vi "UI Error Handler - Main Loop.vi"(1 "Error In":errorcluster, 2 "Message Queue":refnum<queue>) -> ()   [LabVIEW 2017]
uses:
  Support/Message Queue/Message Cluster.ctl
  Support/Message Queue/Message Queue.lvlib
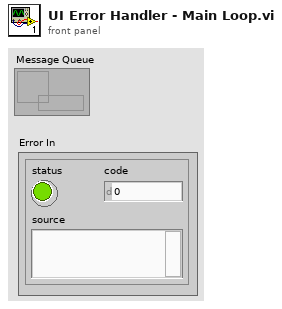
[diagram p1: front panel]
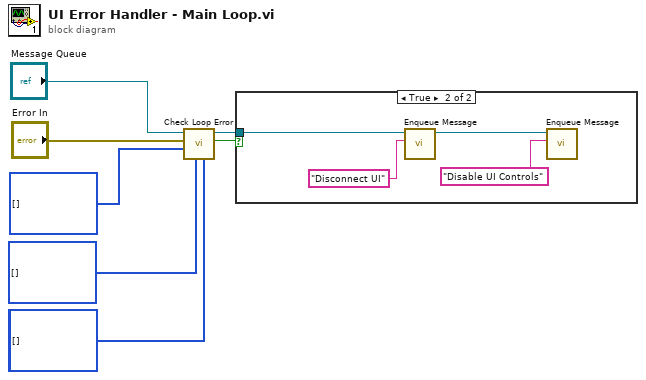
[diagram p0: block diagram]
diagram:
  (unwired) i32[] [] ("Critical Errors")
  n1 = call "Check Loop Error.vi"("Ignore Errors"=i32[] [] ("Critical Errors"), "Log-Only Errors"=i32[] [] ("Critical Errors"), "Critical Errors"=i32[] [], "error to process"="Error In", "Message Queue"="Message Queue") -> ("Enqueued Error?"=w2:bool, "dup Message Queue"=w1:refnum<queue>)  [unwired: 5 in]
  n2 = case shown="True" w2 {
    tunnel: w1 -> [_ w9]
    frame False {
    }
    frame True {
      n3 = call "Enqueue Message.vi"("Message"="Disconnect UI", "Message Queue"=w9) -> ("dup Message Queue"=w10:refnum<queue>)  [unwired: 8 in, 1 out]
      n4 = call "Enqueue Message.vi"("Message"="Disable UI Controls", "Message Queue"=w10) -> ()  [unwired: 8 in, 2 out]
    }
  }
